vi "Reconnect To Target.vi"(8 "Error In":errorcluster, 11 "Install LV Data in":T1) -> (0 "Error Out":errorcluster, 2 "Connected?":bool, 3 "Install LV Data out":T1)   [LabVIEW 2014, in "LMH-LINX.lvlib"]
uses:
  <vilib>/MakerHub/LINX/LMH-LINX.lvlib
  <vilib>/MakerHub/LINX/Private/Utilties/Target Management/Install LV Data.ctl
  C:/Program Files (x86)/National Instruments/LabVIEW 2014/vi.lib/MakerHub/LINX/Resources/Renci.SshNet.dll
  Resources/Renci.SshNet.dll
  <vilib>/MakerHub/LINX/Private/Utilties/Target Management/Target Info.ctl
  <vilib>/MakerHub/LINX/Private/Utilties/Target Management/NIC Info.ctl
  <vilib>/MakerHub/LINX/Private/Utilties/Target Management/NIC Mode.ctl
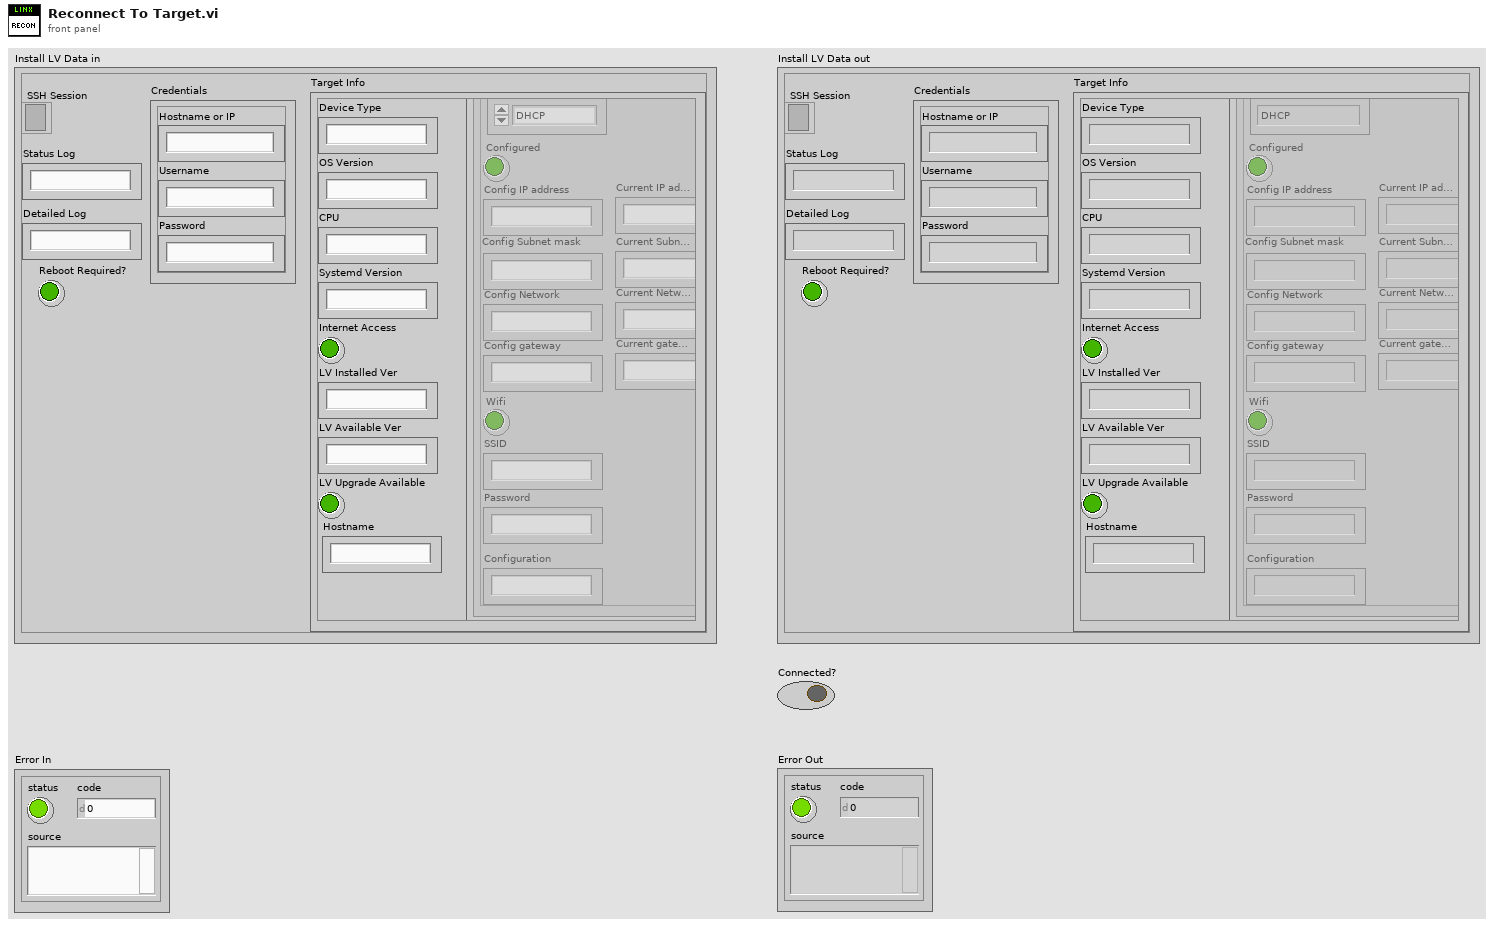
[diagram p1: front panel]
types:
  T1 = typedef "LMH-LINX.lvlib/Install LV Data.ctl" = cluster{"SSH Session":refnum<k24>, "Status Log":string, "Detailed Log":string, "Credentials":cluster{"Hostname or IP":string, "Username":string, "Password":string}, "Target Info":T2, "Reboot Required?":bool}
  T2 = typedef "LMH-LINX.lvlib/Target Info.ctl" = cluster{"OS Version":string, "CPU":string, "Systemd Version":string, "Internet Access":bool, "Device Type":string, "LV Installed Ver":string, "LV Available Ver":string, "LV Upgrade Available":bool, "Hostname":string, "NIC Info":T3[]}
  T3 = typedef "LMH-LINX.lvlib/NIC Info.ctl" = cluster{"Name":string, "NIC Mode":T4, "Configured":bool, "Config IP address":string, "Config Subnet mask":string, "Config Network":string, "Config gateway":string, "Wifi":bool, "SSID":string, "Password":string, "Configuration":string, "Current IP address":string, "Current Subnet mask":string, "Current gateway":string, "Current Network":string}
  T4 = typedef "LMH-LINX.lvlib/NIC Mode.ctl" = enum16{"DHCP", "Static", "Loopback"}
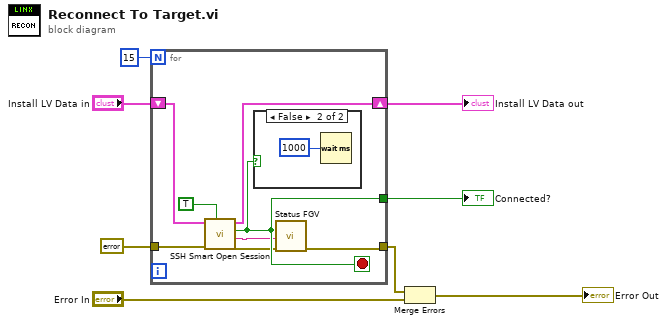
[diagram p0: block diagram]
diagram:
  n1 = for {
    N: 15 -> [_]
    tunnel: errorcluster {"status"=FALSE, "code"=0, "source"=""} ("Error Out") -> [w16]
    shift-right: [w13] -> w5
    shift-left: "Install LV Data in" -> [w15]
    tunnel: [w10] -> w3
    tunnel: [w12] -> w7
    stop <- w12 stop-if-true
    n2 = call <vilib>:"SSH Smart Open Session.vi"("Force Reconnect?"=TRUE, "Error In"=w16, "Install LV Data in"=w15) -> ("Error Out"=w11:errorcluster, "Status"=w9:string, "Connected?"=w12:bool, "Install LV Data out"=w13:T1)  [unwired: 5 in]
    n3 = case shown="False" w12 {
      frame True {
      }
      frame False {
        n4 = Wait (ms)(milliseconds to wait=u32 1000) -> ()  [unwired: 1 out]
      }
    }
    n5 = call <vilib>:"Status FGV.vi"("Error In"=w11, "Status"=w9) -> ("Error Out"=w10:errorcluster)  [unwired: 7 in, 2 out]
  }
  "Connected?" <- w7
  "Install LV Data out" <- w5
  n6 = Merge Errors(w3, "Error In") -> (→"Error Out":errorcluster)
